vi "ZK加标体积读取.vi"(7 "是否启用通讯通知":bool, 8 "error in (no error)":errorcluster, 11 "Slave ID":T1) -> (0 "error out":errorcluster, 3 "加标体积":sgl)   [LabVIEW 2016, in "质控单元V4.lvlib"]
uses:
  <vilib>/Plasmionique/MB Master/MB_Master/MB_Master.lvclass
  <vilib>/Plasmionique/MB Master/MB Master.lvlib
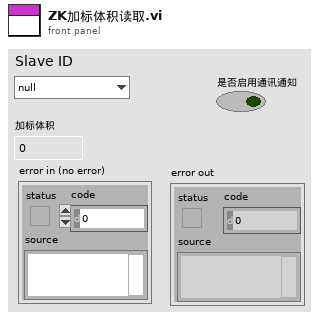
[diagram p1: front panel]
types:
  T1 = typedef "质控单元V4.lvlib/质控slave id.ctl" = enum16{"null", "氨氮", "总磷", "总氮", "CODMn", "CODCr", "氟化物", "挥发酚"}
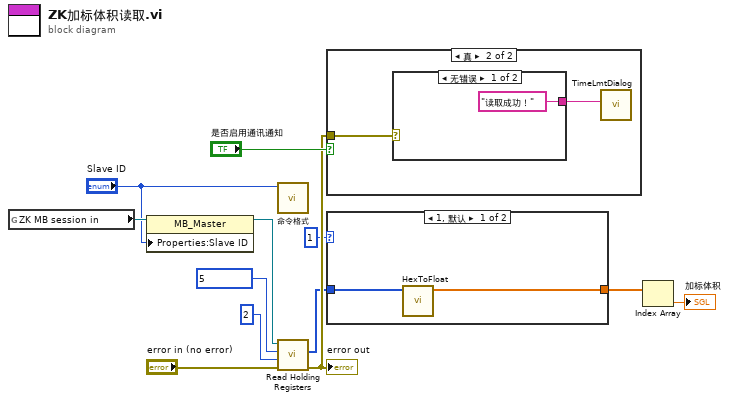
[diagram p0: block diagram]
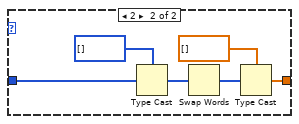
[diagram p2: hidden frame]
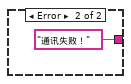
[diagram p4: hidden frame]
diagram:
  n1 = global read "ZK非断电保存全局变量.vi" "ZK MB session in"() -> (w11:refnum<class "MB_Master.lvclass">)
  n2 = property class="MB_Master"(reference=w11, "Properties:Slave ID"="Slave ID") -> (reference out=w9:refnum<class "MB_Master.lvclass">)  [unwired: 1 in, 1 out]
  n3 = call "命令格式.vi"("Slave ID"="Slave ID") -> ()  [unwired: 10 in, 1 out]
  n4 = call <vilib>:"Read Holding Registers.vi"("error in (no error)"="error in (no error)", "quantity"=u16 2, "starting address"=u16 5, "MB session in"=w9) -> ("error out"=w5:errorcluster, "Registers"=w4:u16[])  [unwired: 5 in, 1 out]
  "error out" <- w5
  n5 = case shown="真" "是否启用通讯通知" {
    tunnel: w5 -> [_ w14]
    frame False {
    }
    frame True {
      n6 = case shown="无错误" w14 {
        tunnel: ["读取成功！" "通讯失败！"] -> w13
        frame No Error {
        }
        frame Error {
        }
      }
      n7 = call "TimeLmtDialog.vi"("Infoin"=w13) -> ()  [unwired: 11 in]
    }
  }
  n8 = case shown="1, 默认" u16 1 ("CODCr 命令格式 in") {
    tunnel: w4 -> [w18 w21]
    tunnel: [w17 w23] -> w3
    frame 1, Default {
      n9 = call "HexToFloat.vi"("数组"=w18) -> ("FLOAT"=w17:sgl[])  [unwired: 10 in]
    }
    frame 2 {
      n10 = Type Cast(type=u32[] [], x=w21) -> (*(type *) &x=w20:u32[])
      n11 = Swap Words(1:w20) -> (0:w19:u32[])
      n12 = Type Cast(type=sgl[] [], x=w19) -> (*(type *) &x=w23:sgl[])
    }
  }
  n13 = Index Array(array=w3) -> (element=→"加标体积":sgl)  [unwired: 1 in]
